vi "oa_Get Last Index.vi"(6 "block size":i32=1024 min=2, 9 "trigger indices":T1, 11 "even angle signal":cluster{"r0":dbl, "dr":dbl, "Y":dbl[]}={"r0"=0.0, "dr"=1.0, "Y"=[]} {"r0" format="%.2p"; "dr" format="%.2p"; "Y" format="%.2f"}) -> (0 "current positon":cluster{"rev":dbl, "time":dbl, "RPM":dbl}, 1 "trigger indices for buffer":T1, 2 "rev index":dbl, 4 "index in range":bool)   [LabVIEW 2017, in "SoundVib_OAUtility.lvlib"]
uses:
  <vilib>/addons/Sound and Vibration/Order Analysis/Utility/SoundVib_OAUtility.lvlib
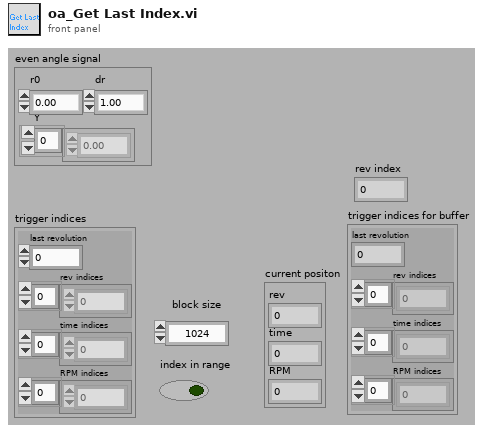
[diagram p1: front panel]
types:
  T1 = cluster{"last revolution":dbl, "rev indices":dbl[], "time indices":dbl[], "RPM indices":dbl[]}
  T2 = cluster{"last revolution":dbl, dbl[], dbl[], dbl[]}
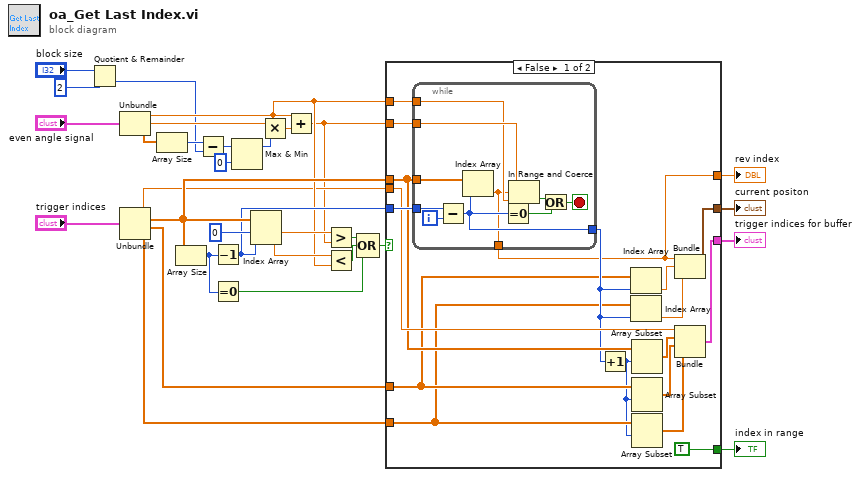
[diagram p0: block diagram]
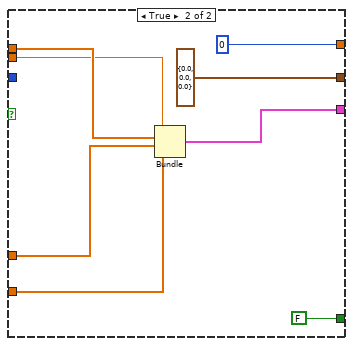
[diagram p2: hidden frame]
diagram:
  n1 = Quotient & Remainder(x="block size", y=2) -> (floor(x/y)=w4:i32)  [unwired: 1 out]
  n2 = Unbundle("even angle signal") -> ("r0"=w21:dbl, "dr"=w29:dbl, "Y"=w30:dbl[])
  n3 = Unbundle("trigger indices") -> ("last revolution"=w11:dbl, "rev indices"=w26:dbl[], "time indices"=w13:dbl[], "RPM indices"=w12:dbl[])
  n4 = Array Size(array=w30) -> (size(s)=w5:i32)
  n5 = Array Size(array=w26) -> (size(s)=w10:i32)
  n6 = Subtract(x=w5, y=w4) -> (x-y=w3:i32)
  n7 = Decrement(x=w10) -> (x-1=w24:i32)
  n8 = Equal To 0?(x=w10) -> (x = 0?=w9:bool)
  n9 = Max & Min(x=w3, y=0) -> (max(x,y)=w2:i32)  [unwired: 1 out]
  n10 = Index Array(array=w26, index #1=0 ("index"), index #2=w24) -> (element #1=w23:dbl, element #2=w22:dbl)
  n11 = Multiply(x=w29, y=w2) -> (x*y=w28:dbl)
  n12 = Add(x=w21, y=w28) -> (x+y=w6:dbl)
  n13 = Greater?(x=w23, y=w6) -> (0:w20:bool)
  n14 = Less?(x=w22, y=w21) -> (x < y?=w19:bool)
  n15 = Compound Arithmetic op=OR(w20, w19, w9) -> (w18:bool)
  n16 = case shown="False" w18 {
    tunnel: [w32 0] -> w27
    tunnel: w26 -> [w41 w64]
    tunnel: w24 -> [w49 _]
    tunnel: w6 -> [w48 _]
    tunnel: w21 -> [w47 _]
    tunnel: [TRUE FALSE] -> w17
    tunnel: [w39 w60] -> w15
    tunnel: [w43 cluster{"rev":dbl, "time":dbl, "RPM":dbl} {"rev"=0.0, "time"=0.0, "RPM"=0.0} ("current positon")] -> w14
    tunnel: w13 -> [w38 w63]
    tunnel: w12 -> [w35 w62]
    tunnel: w11 -> [w42 w61]
    frame False {
      n17 = while {
        tunnel: w41 -> [w59]
        tunnel: w49 -> [w58]
        tunnel: w48 -> [w56]
        tunnel: w47 -> [w55]
        tunnel: [w51] -> w40
        tunnel: [w50] -> w32
        i -> [w57]
        stop <- w52 stop-if-true
        n18 = Subtract(x=w58, y=w57) -> (x-y=w51:i32)
        n19 = Index Array(array=w59, index=w51) -> (element=w50:dbl)
        n20 = Equal To 0?(x=w51) -> (x = 0?=w54:bool)
        n21 = In Range and Coerce(upper limit=w56, x=w50, lower limit=w55) -> (In Range?=w53:bool)  [unwired: 1 out]
        n22 = Or(x=w53, y=w54) -> (x .or. y?=w52:bool)
      }
      n23 = Increment(x=w40) -> (x+1=w34:i32)
      n24 = Index Array(array=w38, index=w40) -> (element=w45:dbl)
      n25 = Index Array(array=w35, index=w40) -> (element=w44:dbl)
      n26 = Array Subset(array=w41, index=w34) -> (w37:dbl[])  [unwired: 1 in]
      n27 = Array Subset(array=w38, index=w34) -> (w36:dbl[])  [unwired: 1 in]
      n28 = Array Subset(array=w35, index=w34) -> (w33:dbl[])  [unwired: 1 in]
      n29 = Bundle(w32, "start"=w45, "start"=w44) -> (w43:cluster{dbl, "start":dbl, "start":dbl})  [unwired: 1 in]
      n30 = Bundle("last revolution"=w42, w37, w36, w33) -> (w39:T2)  [unwired: 1 in]
    }
    frame True {
      n31 = Bundle("last revolution"=w61, "rev indices"=w64, "time indices"=w63, "RPM indices"=w62) -> (w60:T1)  [unwired: 1 in]
    }
  }
  "trigger indices for buffer" <- w15
  "current positon" <- w14
  "rev index" <- w27
  "index in range" <- w17
